vi "Get Forecast Hourly Data.vi"(8 "error in (no error)":errorcluster, 11 "API Output":string) -> (0 "error out":errorcluster, 2 "Hourly Data":T1 {"hourly"."data"."time" format="%#_10g"}, 3 "API Output (copy)":string)   [LabVIEW 2017, in "Dark Sky Weather Data for LabVIEW.lvlib"]
doc: "Parses the Dark Sky API's output for weather data by the hour for the next 48 hours"
uses:
  Dark Sky Weather Data for LabVIEW.lvlib
  Controls/Forecast Hourly Data.ctl
  <vilib>/addons/_JKI.lib/Serialization/JSON/JKI JSON Serialization.lvlib
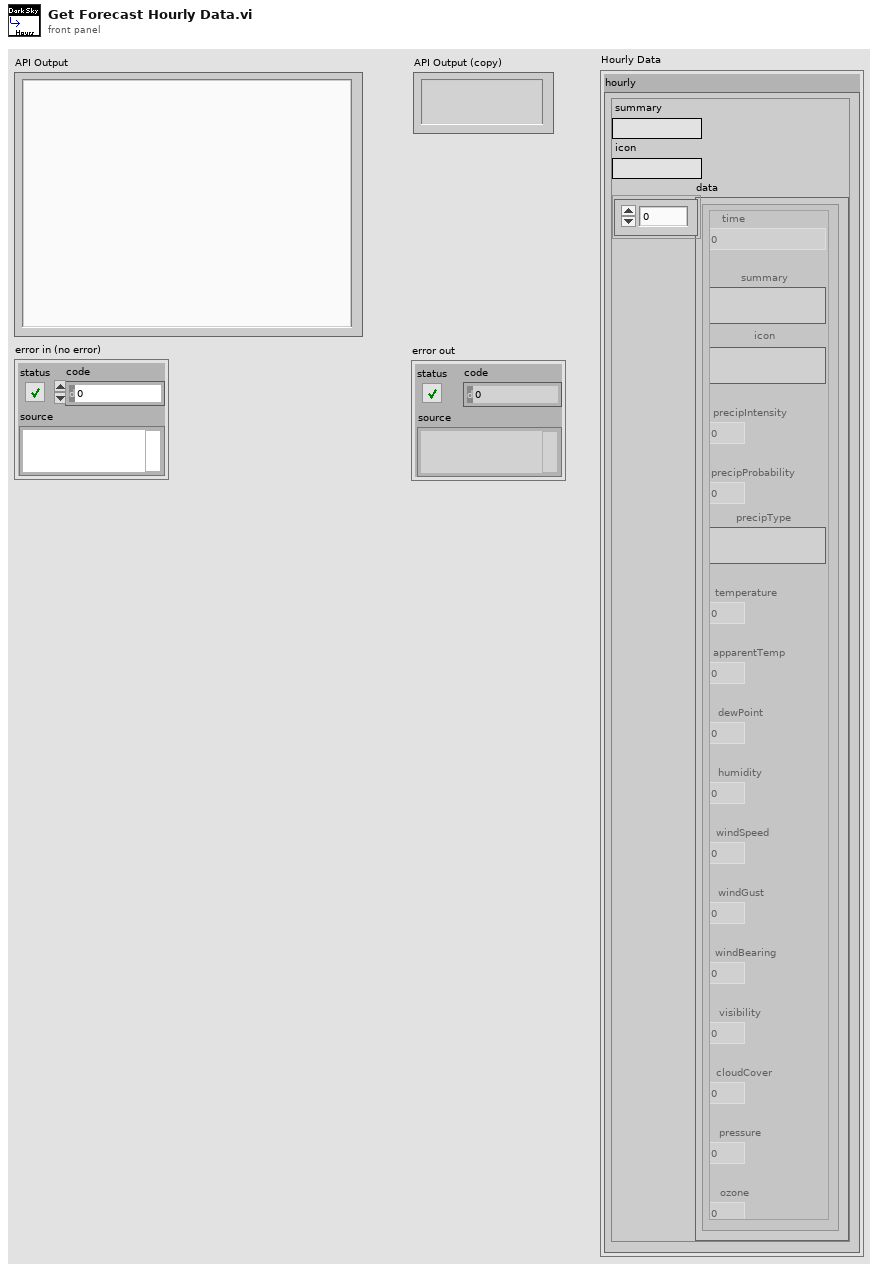
[diagram p1: front panel]
types:
  T1 = typedef "Dark Sky Weather Data for LabVIEW.lvlib/Forecast Hourly Data.ctl" = cluster{"hourly":cluster{"summary":string, "icon":string, "data":cluster{"time":dbl, "summary":string, "icon":string, "precipIntensity":dbl, "precipProbability":dbl, "precipType":string, "temperature":dbl, "apparentTemp":dbl, "dewPoint":dbl, "humidity":dbl, "windSpeed":dbl, "windGust":dbl, "windBearing":dbl, "visibility":dbl, "cloudCover":dbl, "pressure":dbl, "ozone":dbl}[]}}
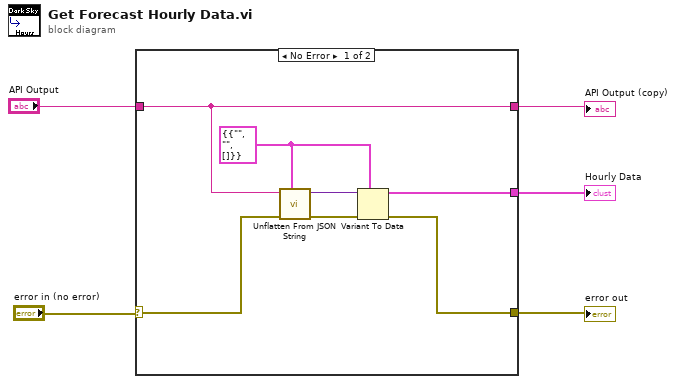
[diagram p0: block diagram]
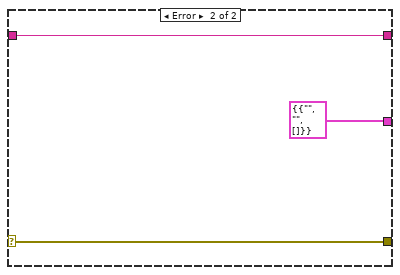
[diagram p2: hidden frame]
diagram:
  n1 = case shown="No Error" "error in (no error)" {
    selector: "error in (no error)" -> [w12 w15]
    tunnel: [w9 w15] -> w4
    tunnel: "API Output" -> [w8 w14]
    tunnel: [w8 w14] -> w2
    tunnel: [w7 T1 {"hourly"={"summary"="", "icon"="", "data"=[]}} ("Hourly Data")] -> w1
    frame No Error {
      w6 = T1 {"hourly"={"summary"="", "icon"="", "data"=[]}} ("Hourly Data")
      n2 = call <vilib>:"Unflatten From JSON String.vi"("Type and Defaults"=w6, "error in (no error)"=w12, "JSON String"=w8) -> ("error out"=w10:errorcluster, "Variant"=w11:variant)  [unwired: 7 in]
      n3 = Variant To Data(error in=w10, type=w6, Variant=w11) -> (data=w7:T1, error out=w9:errorcluster)
    }
    frame Error {
    }
  }
  "error out" <- w4
  "API Output (copy)" <- w2
  "Hourly Data" <- w1
